vi "GetTempN1911a.vi"(3 "error in (no error)":errorcluster) -> (0 "Error out":errorcluster, 1 "String_Temp_n1911a":string, 2 "N1911a Temp (C)":dbl format="%#.10f")   [LabVIEW 2009]
doc: "Reads the temperature from the probe of the N1911A power meter."
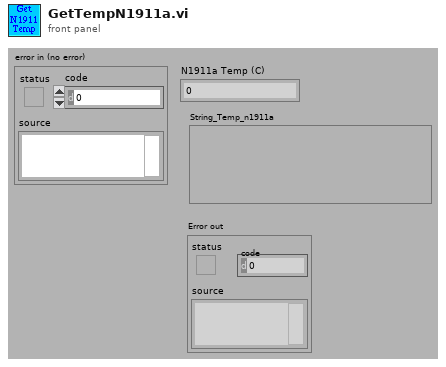
[diagram p1: front panel]
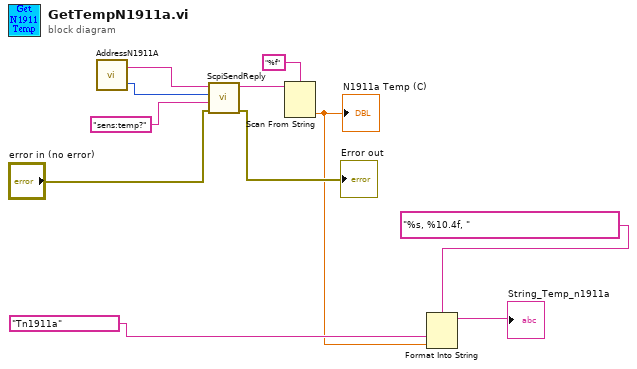
[diagram p0: block diagram]
diagram:
  n1 = call "AddressN1911A.vi"() -> ("Port"=w6:i32, "IP address"=w5:string)  [unwired: 2 in]
  n2 = call "ScpiSendReply.vi"("error in (no error)"="error in (no error)", "Command"="sens:temp?" ("format string"), "TCP port"=w6, "IP Address"=w5) -> ("Error out"=→"Error out":errorcluster, "Reply"=w9:string)  [unwired: 5 in]
  n3 = Scan From String(format string="%f", input string=w9) -> (output 1=w2:dbl)  [unwired: 3 in, 3 out]
  "N1911a Temp (C)" <- w2
  n4 = Format Into String(format string="%s, %10.4f, ", "Tn1911a", w2) -> (resulting string=→"String_Temp_n1911a":string)  [unwired: 2 in, 1 out]
